vi "read_string-2.vi"() -> ()   [LabVIEW 2019]
uses:
  <vilib>/RTI DDS Toolkit/Types/DDS Duration.ctl
  <vilib>/RTI DDS Toolkit/Types/RTI DDS Read Mode.ctl
  <vilib>/RTI DDS Toolkit/VIs/SimpleCreateReader_String.vi
  <vilib>/RTI DDS Toolkit/VIs/Read_String.vi
  <vilib>/RTI DDS Toolkit/VIs/Advanced Create Reader.vi
  <vilib>/RTI DDS Toolkit/VIs/AdvancedCreateReader_String.vi
  <vilib>/RTI DDS Toolkit/Library/LVDDS_library.lvlib
panel:
  out "Data":string
  in  "Domain Id":u32
  in  "y":bool
  in  "Topic Name":string="MyTopic"
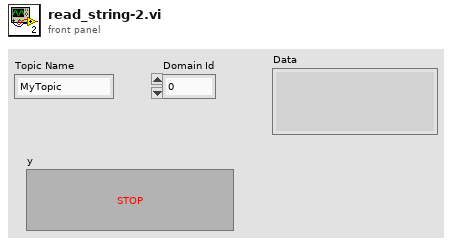
[diagram p1: front panel]
types:
  T1 = typedef "LVDDS_library.lvlib/RTI DDS Read Mode.ctl" = enum32{"LVDDS_READ_MODE_POLLING", "LVDDS_READ_MODE_BLOCKING"}
  T2 = typedef "LVDDS_library.lvlib/DDS Duration.ctl" = cluster{"sec":i32, "nanosec":u32}
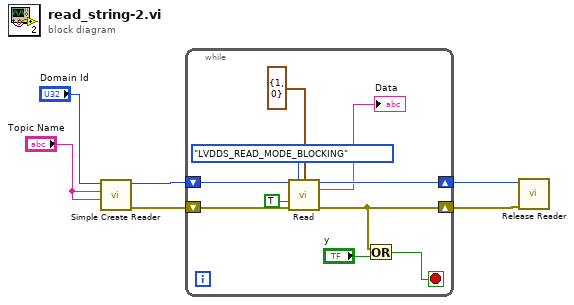
[diagram p0: block diagram]
diagram:
  n1 = call-poly <vilib>:"Simple Create Reader.vi"("Type"="Topic Name", "Topic Name"="Topic Name", "Domain Id"="Domain Id") -> ("error out"=w5:errorcluster, "DDS Object Ref"=w6:u64)  [unwired: 7 in]
  n2 = while {
    shift-right: [w15] -> w1
    shift-left: w6 -> [w16]
    shift-right: [w11] -> w2
    shift-left: w5 -> [w14]
    stop <- w12 stop-if-true
    n3 = call-poly <vilib>:"Read.vi"("DDS Object Ref in"=w16, "Read Mode"=RTI_DDS_Read_Mode."LVDDS_READ_MODE_BLOCKING", "Blocking Timeout"=T2 {"sec"=1, "nanosec"=0}, "Only New Samples"=TRUE, "error in (no error)"=w14) -> ("DDS Object Ref out"=w15:u64, "Data"=→"Data":string, "error out"=w11:errorcluster)  [unwired: 6 in, 2 out]
    n4 = Or(x=w11, y="y") -> (x .or. y?=w12:bool)
  }
  n5 = call <vilib>:"Release Reader.vi"("error in (no error)"=w2, "DDS Object Ref"=w1) -> ()  [unwired: 9 in, 1 out]
